vi "Confirmation_Rumble.vi"(0 "Duration":u32, 1 "Set":bool, 2 "Joystick Refnum Name":string="Pilot Controller") -> ()   [LabVIEW 2018]
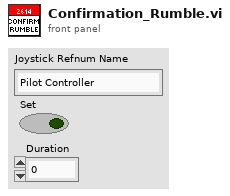
[diagram p1: front panel]
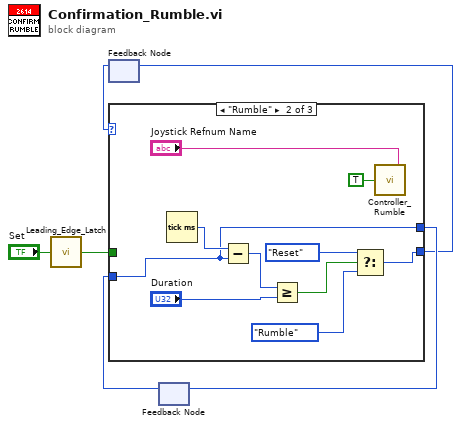
[diagram p0: block diagram]
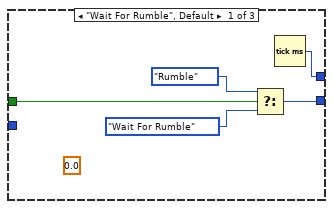
[diagram p2: hidden frame]
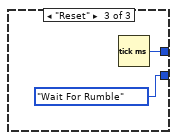
[diagram p3: hidden frame]
diagram:
  n1 = call "Leading_Edge_Latch.vi"("Input"="Set") -> ("Output"=w1:bool)
  n2 = feedback #1() -> (w3:enum16{"Wait For Rumble", "Rumble", "Reset"})  [unwired: 1 in]
  n3 = feedback #2() -> (w5:u32)  [unwired: 1 in]
  n4 = case shown="\"Rumble\"" w3 {
    tunnel: [w11 w12 w23] -> w6
    tunnel: w5 -> [_ w12 _]
    tunnel: [w8 w21 enum16{"Wait For Rumble", "Rumble", "Reset"}."Wait For Rumble" ("f")] -> w4
    tunnel: w1 -> [w7 _ _]
    frame "Wait For Rumble", Default {
      (unwired) 0.0
      n5 = Select(t=enum16{"Wait For Rumble", "Rumble", "Reset"}."Rumble" ("Rumble"), s=w7, f=enum16{"Wait For Rumble", "Rumble", "Reset"}."Wait For Rumble") -> (s? t:f=w8:enum16{"Wait For Rumble", "Rumble", "Reset"})
      n6 = Tick Count (ms)() -> (millisecond timer value=w11:u32)
    }
    frame "Rumble" {
      n7 = Tick Count (ms)() -> (millisecond timer value=w16:u32)
      n8 = Subtract(x=w16, y=w12) -> (x-y=w15:u32)
      n9 = Greater Or Equal?(x=w15, y="Duration") -> (x >= y?=w13:bool)
      n10 = Select(t=enum16{"Wait For Rumble", "Rumble", "Reset"}."Reset" ("f"), s=w13, f=enum16{"Wait For Rumble", "Rumble", "Reset"}."Rumble") -> (s? t:f=w21:enum16{"Wait For Rumble", "Rumble", "Reset"})
      n11 = call "Controller_Rumble.vi"("Joystick Refnum Name"="Joystick Refnum Name", "Rumble"=TRUE) -> ()
    }
    frame "Reset" {
      n12 = Tick Count (ms)() -> (millisecond timer value=w23:u32)
    }
  }
  n13 = feedback-in #1(w4) -> ()
  n14 = feedback-in #2(w6) -> ()
